vi "DTC_READ.vi"(11 "DTC Value":string) -> (3 "DTC Type":string)   [LabVIEW 2020]
uses:
  CheminDeBase.vi
  <vilib>/regexp/Match Regular Expression.xnode
panel:
  out "DTC list":string
  # "820066"
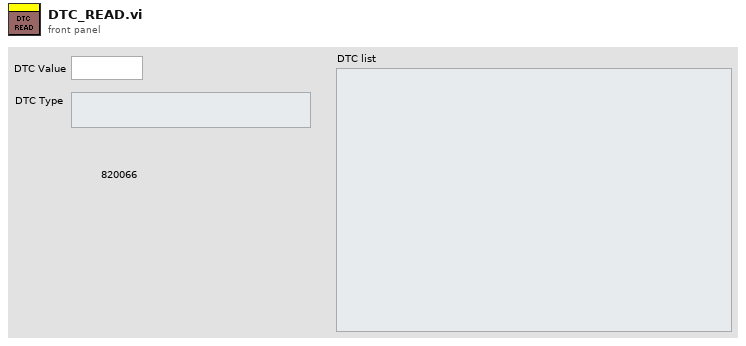
[diagram p1: front panel]
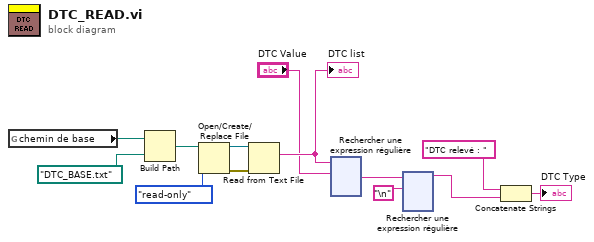
[diagram p0: block diagram]
diagram:
  n1 = global read "CheminDeBase.vi" "chemin de base"() -> (w13:path)
  n2 = Build Path(base path=w13, name or relative path=path "DTC_BASE.txt" ("nom ou chemin relatif")) -> (appended path=w11:path)
  n3 = Open/Create/Replace File(file path (use dialog)=w11, access (0:read/write)=enum16{"read/write", "read-only", "write-only"}."read-only" ("accès (0 : read/write)")) -> (refnum out=w9:refnum<file>, error out=w8:errorcluster)  [unwired: 4 in, 1 out]
  n4 = Read from Text File(file (use dialog)=w9, error in=w8) -> (text=w7:string)  [unwired: 2 in, 3 out]
  "DTC list" <- w7
  n5 = xnode "Rechercher une expression régulière"("chaîne en entrée"=w7, "expression régulière"="DTC Value") -> ("après la correspondance"=w5:string)  [unwired: 4 in, 4 out]
  n6 = xnode "Rechercher une expression régulière"("chaîne en entrée"=w5, "expression régulière"="\n") -> ("avant la correspondance"=w3:string)  [unwired: 4 in, 4 out]
  n7 = Concatenate Strings("DTC relevé : " ("chaîne"), w3) -> (→"DTC Type":string)
